vi "U6 LJTDAC Single Channel Example.vi"() -> (0 "error out":errorcluster)   [LabVIEW 2021]
panel:
  in  "DAC A?":bool=TRUE
  in  "DAC Value":dbl step=0.01 format="%.4f"
  in  "FirstFound":bool=TRUE
  in  "Address":string="1"
  out "Error Message":string
  in  "SCL Pin #":i32
  # "Update a channel on an LJTick-DAC."
  # "A\n\nB"
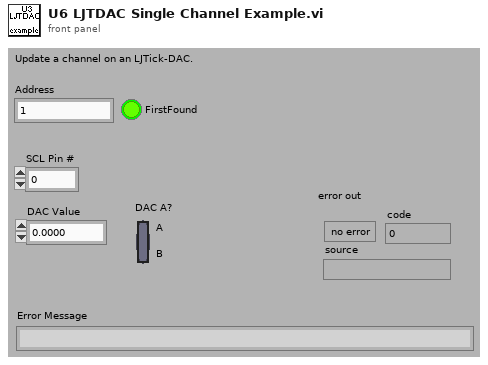
[diagram p1: front panel]
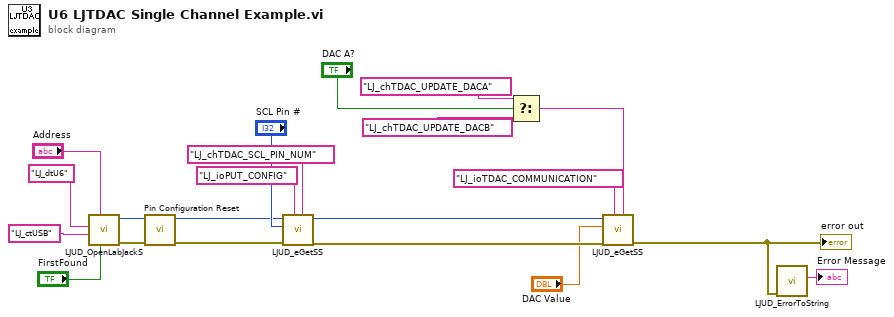
[diagram p0: block diagram]
diagram:
  n1 = call "LJUD_OpenLabJackS.vi"("FirstFound"="FirstFound", "Address"="Address", "ConnectionType"="LJ_ctUSB", "DeviceType"="LJ_dtU6") -> ("error out"=w15:errorcluster, "Handle"=w16:i32)  [unwired: 5 in, 1 out]
  n2 = call "Pin Configuration Reset.vi"("error in"=w15, "Handle In"=w16) -> ("error out"=w10:errorcluster, "Handle Out"=w11:i32)  [unwired: 8 in]
  n3 = call "LJUD_eGetSS.vi"("Channel"="LJ_chTDAC_SCL_PIN_NUM", "IOType"="LJ_ioPUT_CONFIG", "error in"=w10, "Value Write"="SCL Pin #", "Handle In"=w11) -> ("error out"=w7:errorcluster, "Handle Out"=w8:i32)  [unwired: 4 in, 1 out]
  n4 = Select(t="LJ_chTDAC_UPDATE_DACA" ("Channel"), s="DAC A?", f="LJ_chTDAC_UPDATE_DACB" ("Channel")) -> (s? t:f=w2:string)
  n5 = call "LJUD_eGetSS.vi"("Channel"=w2, "IOType"="LJ_ioTDAC_COMMUNICATION", "error in"=w7, "Value Write"="DAC Value", "Handle In"=w8) -> ("error out"=w1:errorcluster)  [unwired: 4 in, 2 out]
  "error out" <- w1
  n6 = call "LJUD_ErrorToString.vi"("error in"=w1) -> ("String"=→"Error Message":string)  [unwired: 10 in]
